vi "Read Parameters to process.vi"(8 "error in":errorcluster, 11 "GPIC ScaleAndLimit runtime in":refnum<class "GPIC ScaleAndLimit runtime.lvclass">) -> (0 "error out":errorcluster, 2 "Parameters to process":T1, 3 "GPIC ScaleAndLimit runtime out":refnum<class "GPIC ScaleAndLimit runtime.lvclass">)   [LabVIEW 2015, in "GPIC ScaleAndLimit runtime.lvclass"]
uses:
  GPIC ScaleAndLimit runtime.lvclass
  configuration/parameter data indices.ctl
  GPIC ScaleAndLimit runtime.lvclass/GPIC ScaleAndLimit runtime.ctl
  configuration/GPIC ScaleAndLimit configuration.lvclass
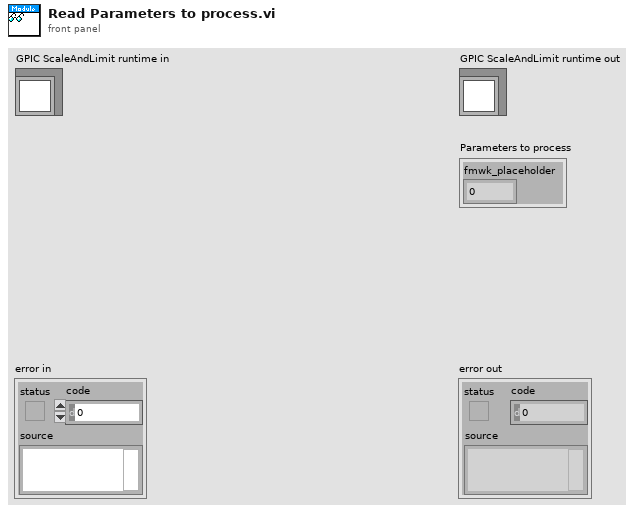
[diagram p1: front panel]
types:
  T1 = typedef "GPIC ScaleAndLimit configuration.lvclass/parameter data indices.ctl" = cluster{"fmwk_placeholder":i32}
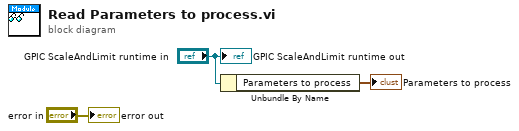
[diagram p0: block diagram]
diagram:
  n1 = Unbundle By Name("GPIC ScaleAndLimit runtime in") -> ("Parameters to process"=→"Parameters to process":T1)
  "error out" <- "error in"
  "GPIC ScaleAndLimit runtime out" <- "GPIC ScaleAndLimit runtime in"
